vi "Move Forward.vi"(5 "Facing Direction":T1, 6 "Current Position":i32, 9 "Facing Road in":T2[](array[typedef]) items=["Empty", "Portal", "Open", "Wall", ">", "<", ">-^", ">-v", "^-<", "v-<"]) -> (0 "Next Position":i32, 3 "Facing Road out":T2[](array[typedef]) items=["Empty", "Portal", "Open", "Wall", ">", "<", ">-^", ">-v", "^-<", "v-<"], 4 "Hit the Wall ?":bool)   [LabVIEW 2020, in "AoC 2022.lvlib"]
uses:
  AoC 2022.lvlib
  Map Tile.ctl
  b0e690e2-d4fb-4732-909d-20a37dfd1b3b.vi
  Map Direction.ctl
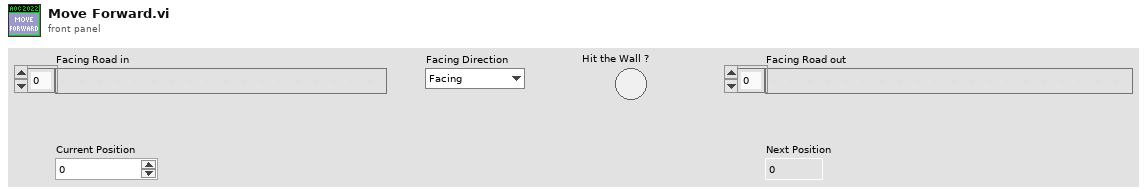
[diagram p1: front panel]
types:
  T1 = typedef "AoC 2022.lvlib/Map Direction.ctl" = enum16{"Facing", "Right", "Left", "Up", "Down"}
  T2 = typedef "AoC 2022.lvlib/Map Tile.ctl" = u16
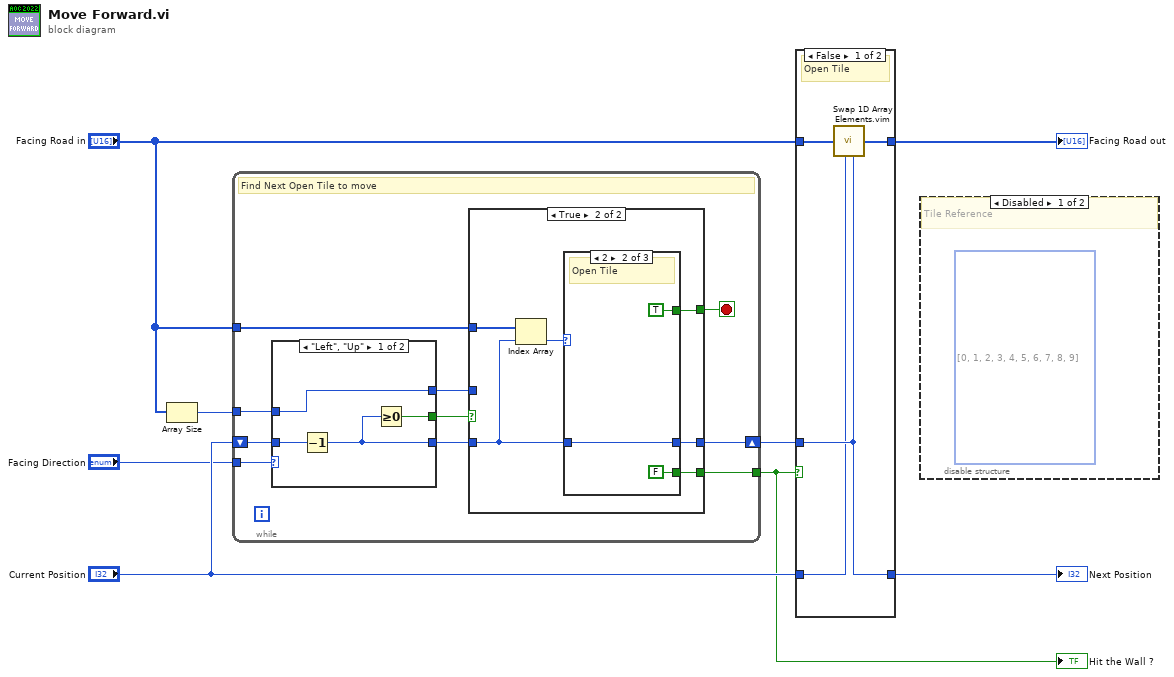
[diagram p0: block diagram]
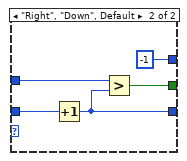
[diagram p2: hidden frame]
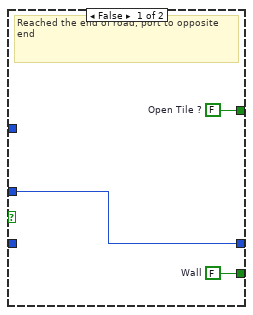
[diagram p3: hidden frame]
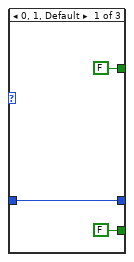
[diagram p4: hidden frame]
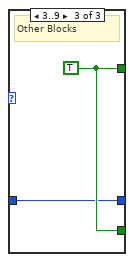
[diagram p5: hidden frame]
diagram:
  n1 = Array Size(array="Facing Road in") -> (size(s)=w5:i32)
  n2 = while {
    tunnel: "Facing Road in" -> [w17]
    shift-right: [w11] -> w3
    shift-left: "Current Position" -> [w18]
    tunnel: w5 -> [w16]
    tunnel: [w12] -> w2
    tunnel: "Facing Direction" -> [w10]
    stop <- w13 stop-if-true
    # "Find Next Open Tile to move"
    n3 = case shown="\"Left\", \"Up\"" w10 {
      tunnel: w18 -> [w22 w27]
      tunnel: w16 -> [w21 w26]
      tunnel: [w20 w25] -> w15
      tunnel: [w19 w24] -> w14
      tunnel: [w21 -1] -> w9
      frame "Left", "Up" {
        n4 = Decrement(x=w22) -> (x-1=w20:i32)
        n5 = Greater Or Equal To 0?(x=w20) -> (x >= 0?=w19:bool)
      }
      frame "Right", "Down", Default {
        n6 = Increment(x=w27) -> (x+1=w25:i32)
        n7 = Greater?(x=w26, y=w25) -> (0:w24:bool)
      }
    }
    n8 = case shown="True" w14 {
      tunnel: w17 -> [_ w36]
      tunnel: w15 -> [_ w31]
      tunnel: [w30 w34] -> w13
      tunnel: [w29 w33] -> w12
      tunnel: [w28 w32] -> w11
      tunnel: w9 -> [w28 _]
      frame False {
        w29 = FALSE  # Wall
        w30 = FALSE  # Open Tile ?
        # "Reached the end of road, port to opposite end"
      }
      frame True {
        n9 = Index Array(array=w36, index=w31) -> (element=w35:T2)
        n10 = case shown="2" w35 {
          tunnel: [FALSE TRUE w44] -> w34
          tunnel: [FALSE FALSE w44] -> w33
          tunnel: [w37 w40 w43] -> w32
          tunnel: w31 -> [w37 w40 w43]
          frame 0, 1, Default {
          }
          frame 2 {
            # "Open Tile"
          }
          frame 3..9 {
            w44 = TRUE
            # "Other Blocks"
          }
        }
      }
    }
  }
  "Hit the Wall ?" <- w2
  n11 = case shown="False" w2 {
    tunnel: [w48 w50] -> w8
    tunnel: "Current Position" -> [w45 w49]
    tunnel: "Facing Road in" -> [w47 w50]
    tunnel: w3 -> [w46 _]
    tunnel: [w46 w49] -> w4
    frame False {
      # "Open Tile"
      n12 = call "Swap 1D Array Elements.vim"("Array in"=w47, "Index 1"=w45, "Index 2"=w46) -> ("Array out"=w48:T2[])
    }
    frame True {
      # "Wall"
    }
  }
  "Facing Road out" <- w8
  "Next Position" <- w4
  n13 = disable-structure shown="Disabled" {
    frame Disabled {
      (unwired) T2[] [0, 1, 2, 3, 4, 5, 6, 7, 8, 9] items=["Empty", "Portal", "Open", "Wall", ">", "<", ">-^", ">-v", "^-<", "v-<"]
      # "Tile Reference"
    }
    frame Enabled {
    }
  }
